vi "Overlay Circle (Center, Radius).vi"(4 "Drawing Mode (Frame)":u32(ring)=1 items=["Frame", "Fill"], 6 "Color":u32(colorbox), 7 "Overlay Group":string, 8 "error in (no error)":errorcluster, 9 "Radius":i32, 10 "Center":T1 {"Y" format="%.2f"; "X" format="%.2f"}, 11 "Image Refnum in":T2) -> (0 "error out":errorcluster, 3 "Image Refnum out":T2)   [LabVIEW 2021, in "Image.lvlib"]
uses:
  Image.lvlib
  <vilib>/vision/Image Controls.llb/IMAQ Image.ctl
panel:
  # "see the AlliGator License on the block diagram (Ctrl+E or Window:Show Block Diagram)"
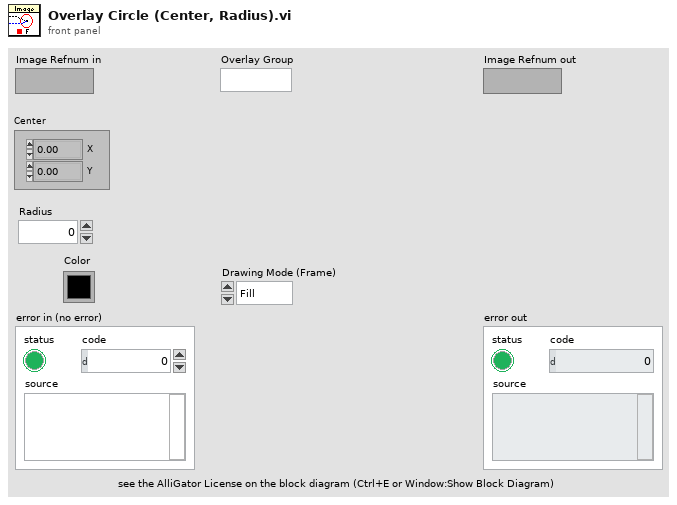
[diagram p1: front panel]
types:
  T1 = typedef "IMAQ Point" = cluster{"X":sgl, "Y":sgl}
  T2 = typedef "IMAQ Image.ctl" = refnum<image>
  T3 = cluster{"Left":i32, "Top":i32, "Right":i32, "Bottom":i32}
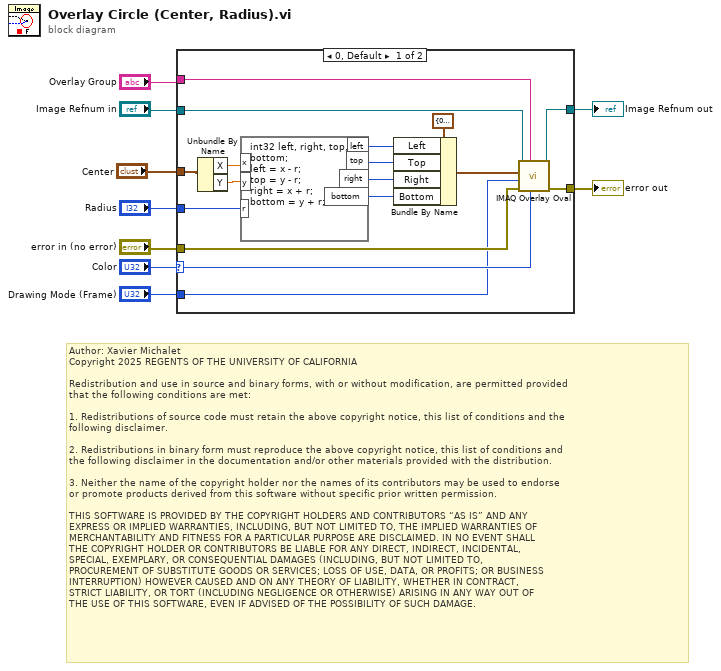
[diagram p0: block diagram]
diagram:
  # "Author: Xavier Michalet\nCopyright 2025 REGENTS OF THE UNIVERSITY OF CALIFORNIA\n\nRedistribution and use in source and binary forms, with or without modification, are permitted provided\nthat the following conditions are met:\n\n1. Redistributions of source code must retain the above copyright notice, this list of conditions and the\nfollowing disclaimer.\n\n2. Redistributions in binary form must reproduce the above copyright notice, this list of conditions and\nthe following disclaimer in the documentation and/or other materials provided with the distribution.\n\n3. Neither the name of the copyright holder nor the names of its contributors may be used to endorse \nor promote products derived from this software without specific prior written permission.\n\nTHIS SOFTWARE IS PROVIDED BY THE COPYRIGHT HOLDERS AND CONTRIBUTORS “AS IS” AND ANY \nEXPRESS OR IMPLIED WARRANTIES, INCLUDING, BUT NOT LIMITED TO, THE IMPLIED WARRANTIES OF\nMERCHANTABILITY AND FITNESS FOR A PARTICULAR PURPOSE ARE DISCLAIMED. IN NO EVENT SHALL\nTHE COPYRIGHT HOLDER OR CONTRIBUTORS BE LIABLE FOR ANY DIRECT, INDIRECT, INCIDENTAL, \nSPECIAL, EXEMPLARY, OR CONSEQUENTIAL DAMAGES (INCLUDING, BUT NOT LIMITED TO, \nPROCUREMENT OF SUBSTITUTE GOODS OR SERVICES; LOSS OF USE, DATA, OR PROFITS; OR BUSINESS\nINTERRUPTION) HOWEVER CAUSED AND ON ANY THEORY OF LIABILITY, WHETHER IN CONTRACT, \nSTRICT LIABILITY, OR TORT (INCLUDING NEGLIGENCE OR OTHERWISE) ARISING IN ANY WAY OUT OF\nTHE USE OF THIS SOFTWARE, EVEN IF ADVISED OF THE POSSIBILITY OF SUCH DAMAGE."
  n1 = case shown="0, Default" "Color" {
    selector: "Color" -> [w26 _]
    tunnel: "Overlay Group" -> [w25 _]
    tunnel: "Image Refnum in" -> [w24 w28]
    tunnel: [w21 w28] -> w5
    tunnel: "error in (no error)" -> [w20 w27]
    tunnel: [w19 w27] -> w7
    tunnel: "Radius" -> [w14 _]
    tunnel: "Drawing Mode (Frame)" -> [w13 _]
    tunnel: "Center" -> [w12 _]
    frame 0, Default {
      n2 = Unbundle By Name(w12) -> ("X"=w11:sgl, "Y"=w10:sgl)
      n3 = formula code="int32 left, right, top, bottom;\nleft = x - r;\ntop = y - r;\nright = x + r;\nbottom = y + r;"("x"=w11, "y"=w10, "r"=w14) -> ("left"=w18:i32, "top"=w17:i32, "right"=w16:i32, "bottom"=w15:i32)
      n4 = Bundle By Name(cluster=T3 {"Left"=0, "Top"=0, "Right"=0, "Bottom"=0} ("Bounding Rectangle"), "Left"=w18, "Top"=w17, "Right"=w16, "Bottom"=w15) -> (w22:T3)
      n5 = call "IMAQ Overlay Oval"("Color"=w26, "Group"=w25, "error in (no error)"=w20, "Drawing Mode (Frame)"=w13, "Bounding Rectangle"=w22, "Image"=w24) -> ("error out"=w19:errorcluster, "Image Out"=w21:T2)  [unwired: 4 in]
    }
    frame 16777216 {
      # "transparent"
    }
  }
  "error out" <- w7
  "Image Refnum out" <- w5
